vi "Sort Wash Options.vi"(11 "Wash Options":T1) -> (3 "Sorted Wash":T2(array[ring]))   [LabVIEW 2017]
uses:
  Controls/Wash Options.ctl
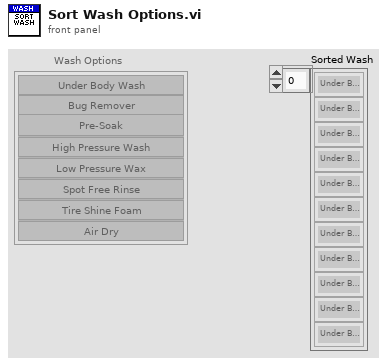
[diagram p1: front panel]
types:
  T1 = typedef "Wash Options.ctl" = cluster{"Underbody Wash":bool, "Bug Remover":bool, "Pre-Soak":bool, "High Pressure Wash":bool, "Low Pressure Wax":bool, "Spot Free Rinse":bool, "Tire Shine Foam":bool, "Air Dry":bool}
  T2 = enum16{"Under Body Wash", "Bug Remover", "Pre-Soak", "High Pressure Wash", "Low Pressure Wax", "Spot Free Rinse", "Tire Shine Foam", "Air Dry", "Skip"}[]
  T3 = enum16{"Under Body Wash", "Bug Remover", "Pre-Soak", "High Pressure Wash", "Low Pressure Wax", "Spot Free Rinse", "Tire Shine Foam", "Air Dry", "Skip"}
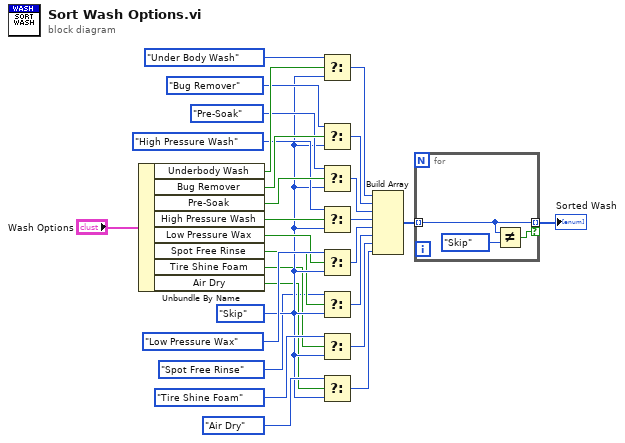
[diagram p0: block diagram]
diagram:
  w16 = T3."Skip"
  n1 = Unbundle By Name("Wash Options") -> ("Underbody Wash"=w28:bool, "Bug Remover"=w26:bool, "Pre-Soak"=w25:bool, "High Pressure Wash"=w22:bool, "Low Pressure Wax"=w17:bool, "Spot Free Rinse"=w15:bool, "Tire Shine Foam"=w14:bool, "Air Dry"=w13:bool)
  n2 = Select(t=T3."Under Body Wash", s=w28, f=w16) -> (s? t:f=w11:T3)
  n3 = Select(t=T3."Bug Remover", s=w26, f=w16) -> (s? t:f=w10:T3)
  n4 = Select(t=T3."Pre-Soak", s=w25, f=w16) -> (s? t:f=w9:T3)
  n5 = Select(t=T3."High Pressure Wash", s=w22, f=w16) -> (s? t:f=w8:T3)
  n6 = Select(t=T3."Low Pressure Wax", s=w17, f=w16) -> (s? t:f=w7:T3)
  n7 = Select(t=T3."Spot Free Rinse", s=w15, f=w16) -> (s? t:f=w6:T3)
  n8 = Select(t=T3."Tire Shine Foam", s=w14, f=w16) -> (s? t:f=w5:T3)
  n9 = Select(t=T3."Air Dry", s=w13, f=w16) -> (s? t:f=w4:T3)
  n10 = Build Array(w11, w10, w9, w8, w7, w6, w5, w4) -> (w3:T2)
  n11 = for {
    tunnel: w3 -> [w30] mode=indexing
    tunnel: [w30] -> w2 mode=indexing if=w29
    n12 = Not Equal?(x=w30, y=T3."Skip") -> (x != y?=w29:bool)
  }
  "Sorted Wash" <- w2
